vi "niRFUtil WFM Pad Waveform with Zeros (complex wfm).vi"(0 "Complex Waveform In":T1 {"y" format="%.2f"; "dx" format="%^.2e"; "x0" format="%^.2e"}, 5 "Required Pre-Trigger Time (s)":dbl, 7 "Required Waveform Duration (s)":dbl=-inf) -> (4 "Complex Waveform Out":T1 {"y" format="%.2f"; "dx" format="%^.2e"; "x0" format="%^.2e"})   [LabVIEW 2015, in "niRFUtil.lvlib"]
uses:
  niRFUtil.lvlib
  Includes/niRFUtil INC Complex Waveform.ctl
  Includes/niRFUtil INC Complex Array.ctl
  Measurements/niRFUtil MEAS Waveform Statistics (complex wfm).vi
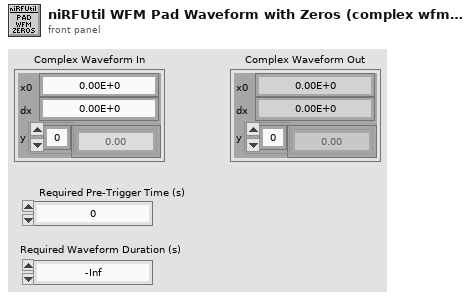
[diagram p1: front panel]
types:
  T1 = typedef "niRFUtil.lvlib/niRFUtil INC Complex Waveform.ctl" = cluster{"x0":dbl, "dx":dbl, "y":T2}
  T2 = typedef "niRFUtil.lvlib/niRFUtil INC Complex Array.ctl" = csg[]
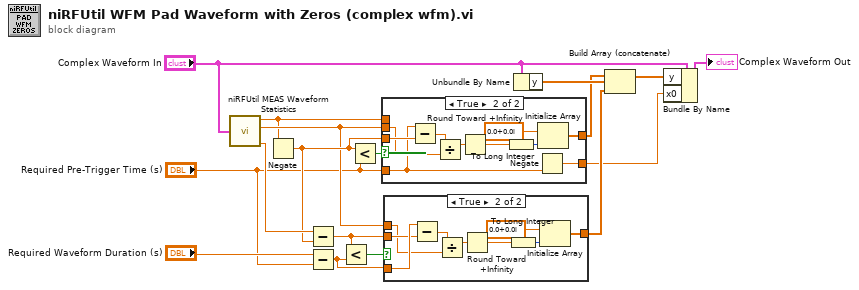
[diagram p0: block diagram]
diagram:
  n1 = call-poly "niRFUtil MEAS Waveform Statistics.vi"("Waveform In"="Complex Waveform In") -> ("Start"=w1:dbl, "Interval"=w9:dbl, "Duration"=w13:dbl)  [unwired: 4 in, 1 out]
  n2 = Negate(x=w1) -> (-x=w12:dbl)
  n3 = Subtract(x=w13, y=w12) -> (x-y=w7:dbl)
  n4 = Subtract(x="Required Waveform Duration (s)", y="Required Pre-Trigger Time (s)") -> (x-y=w8:dbl)
  n5 = Less?(x=w7, y=w8) -> (x < y?=w10:bool)
  n6 = Less?(x=w12, y="Required Pre-Trigger Time (s)") -> (x < y?=w15:bool)
  n7 = case shown="True" w15 {
    tunnel: [_ w27] -> w16
    tunnel: "Required Pre-Trigger Time (s)" -> [_ w20]
    tunnel: w12 -> [_ w26]
    tunnel: w9 -> [_ w24]
    tunnel: [w18 w19] -> w2
    tunnel: w1 -> [w18 _]
    frame False {
    }
    frame True {
      n8 = Subtract(x=w20, y=w26) -> (x-y=w25:dbl)
      n9 = Divide(x=w25, y=w24) -> (x/y=w23:dbl)
      n10 = Round Toward +Infinity(x=w23) -> (ceil(x): smallest int >= x=w22:dbl)
      n11 = To Long Integer(number=w22) -> (32bit integer=w21:i32)
      n12 = Negate(x=w20) -> (-x=w19:dbl)
      n13 = Initialize Array(csg 0.0+0.0i ("element"), w21) -> (w27:csg[])
    }
  }
  n14 = case shown="True" w10 {
    tunnel: [_ w36] -> w14
    tunnel: w8 -> [_ w35]
    tunnel: w7 -> [_ w34]
    tunnel: w9 -> [_ w32]
    frame False {
    }
    frame True {
      n15 = Subtract(x=w35, y=w34) -> (x-y=w33:dbl)
      n16 = Divide(x=w33, y=w32) -> (x/y=w31:dbl)
      n17 = Round Toward +Infinity(x=w31) -> (ceil(x): smallest int >= x=w30:dbl)
      n18 = To Long Integer(number=w30) -> (32bit integer=w29:i32)
      n19 = Initialize Array(csg 0.0+0.0i ("element"), w29) -> (w36:csg[])
    }
  }
  n20 = Unbundle By Name("Complex Waveform In") -> ("y"=w17:T2)
  n21 = Build Array (concatenate)(w16, w17, w14) -> (w5:T2)
  n22 = Bundle By Name(cluster="Complex Waveform In", "y"=w5, "x0"=w2) -> (→"Complex Waveform Out":T1)
